vi "Gasteiler_Endpunkt.vi"   [LabVIEW 2020, in "Linearisierung v2.lvlib"]
uses:
  Linearisierung v2.lvlib
  Gasteiler/Aktionen FGV Gasteiler Daten.ctl
  Gasteiler/AK-Komm Gasteiler/Aktionen AK Komm.ctl
  Gasteiler/AK-Komm Gasteiler/Alter Gasteiler/Aktionen AK Komm_ALT.ctl
  Gasteiler/Horiba/Aktion Befehl.ctl
  Gasteiler/HovaCAL_Interface/Kommunikation/Aktion_FGV_HovaCAL_Interface_SetData.ctl
  Gasteiler/AK-Komm Gasteiler/AK Komm Gasteiler.lvlib
  Gasteiler/Horiba/Horiba GDC.lvlib
  Gasteiler/AK-Komm Gasteiler/Alter Gasteiler/Alter Gasteiler.lvlib
  Gasteiler/Gasteiler.lvlib
  Gasteiler/HovaCAL_Interface/Kommunikation/Kommunikation.lvlib
types:
  T1 = typedef "Linearisierung v2.lvlib/Gasteiler.lvlib/Aktionen FGV Gasteiler Daten.ctl" = enum16{"lesen", "Gasteiler Daten", "Seriellen Param.", "MB-Endwert", "laden", "speichern", "Anforderung", "TCP", "Aufzeichnung Start"}
  T2 = typedef "Linearisierung v2.lvlib/Gasteiler.lvlib/Gasteiler Daten.ctl" = cluster{"Gasteiler":T3, "Gasteiler Stufen":T4, "Gasteiler Type":T5, "Konfig Gasteiler":T6, "Gasteiler Span Eingänge":u16}
  T3 = typedef "String - Eingabefeld.ctl" = string
  T4 = typedef "Linearisierung v2.lvlib/Gasteiler.lvlib/Gasteiler Stufen.ctl" = u16
  T5 = typedef "Linearisierung v2.lvlib/GasteilerType.ctl" = u16
  T6 = typedef "System Einstellungen V2.lvlib/Gasteiler Auswahl.ctl" = u16
  T7 = typedef "Linearisierung v2.lvlib/Gasteiler.lvlib/AK Komm Gasteiler.lvlib/Aktionen AK Komm.ctl" = enum16{"lesen", "initialisieren", "beenden", "Status", "SMAN", "SREM", "STBY", "ASTF", "ASTZ", "SLST", "AGAT", "EGAK", "AGAK", "AKAK", "ADRU", "SKOP", "SVSA", "SVSZ", "SONO", "SAIR", "SNOX", "ANOX", "SSPL", "SRUC", "SLIN", "ALST", "ETYP", "SVIO", "LCYL", "CCYL", "DCYL", "SCYL", "GCYL", "DRGV", "DRDC"}
  T8 = typedef "Linearisierung v2.lvlib/Gasteiler.lvlib/AK Komm Gasteiler.lvlib/Alter Gasteiler.lvlib/Aktionen AK Komm_ALT.ctl" = enum16{"lesen", "initialisieren", "beenden", "SRES", "STBY", "SREM", "SMAN", "SLIN", "SLCH", "SLST", "SSPL", "AGAT", "ALST", "ASTZ", "ASTF", "AGAK", "EGAK"}
  T9 = typedef "Linearisierung v2.lvlib/Gasteiler.lvlib/Horiba GDC.lvlib/Aktion Befehl.ctl" = enum16{"lesen", "initialisieren", "Beenden", "Standby", "GD/CC", "Info", "Flow", "Alarm", "GD parameter", "GD point", "Durchfluss", "Spuelen1", "Spuelen1 On", "Spuelen1Off", "Spuelen2", "Ventil-Abfrage", "Reset"}
  T10 = typedef "Linearisierung v2.lvlib/Gasteiler.lvlib/HovaCAL_Interface.lvlib/Kommunikation.lvlib/Aktion_FGV_HovaCAL_Interface_SetData.ctl" = enum16{"lesen", "Konzentrationen", "Pumpen Parameter", "Pumpe Konzentration", "Pumpe run", "Temperaturen", "Fluss", "Limits", "init"}
  T11 = cluster{"input concentration setpoint":dbl, "output concentration setpoint":dbl}[]
  T12 = cluster{"input concentration setpoint":dbl, "output concentration setpoint":dbl}
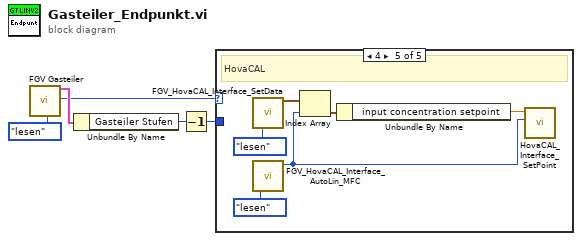
[diagram p0: block diagram]
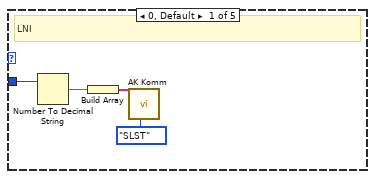
[diagram p2: hidden frame]
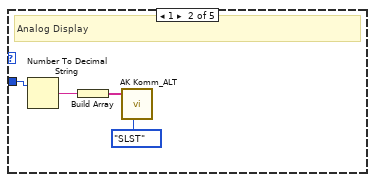
[diagram p3: hidden frame]
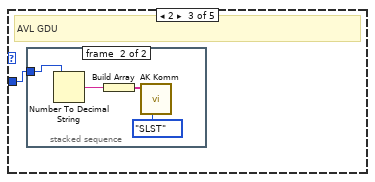
[diagram p4: hidden frame]
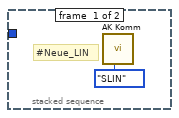
[diagram p5: hidden frame]
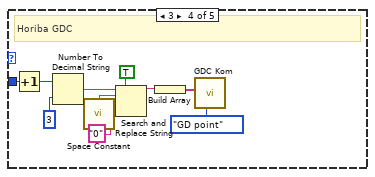
[diagram p6: hidden frame]
diagram:
  n1 = call "FGV Gasteiler.vi"("Aktionen"=Aktionen_FGV_Gasteiler_Daten."lesen") -> ("Gasteiler Daten"=w4:T2, "Gasteiler Type"=w2:T5)  [unwired: 11 in, 6 out]
  n2 = Unbundle By Name(w4) -> ("Gasteiler Stufen"=w1:T4)
  n3 = Decrement(x=w1) -> (x-1=w5:T4)
  n4 = case shown="4" w2 {
    tunnel: w5 -> [w6 w12 w14 w21 _]
    frame 0, Default {
      # "LNI"
      n5 = Number To Decimal String(number=w6) -> (decimal integer string=w9:string)  [unwired: 1 in]
      n6 = Build Array(w9) -> (w8:string[])
      n7 = call "AK Komm.vi"("Aktionen"=Aktionen_AK_Komm."SLST", "Daten"=w8) -> ()  [unwired: 3 in, 7 out]
    }
    frame 1 {
      # "Analog Display"
      n8 = Number To Decimal String(number=w12) -> (decimal integer string=w13:string)  [unwired: 1 in]
      n9 = Build Array(w13) -> (w11:string[])
      n10 = call "AK Komm_ALT.vi"("Aktionen_ALT"=Aktionen_AK_Komm_ALT."SLST", "Daten"=w11) -> ()  [unwired: 5 in, 5 out]
    }
    frame 2 {
      # "AVL GDU"
      n11 = stacked-sequence {
        tunnel: w14 -> [_ w18]
        frame #0 {
          # "#Neue_LIN"
          n12 = call "AK Komm.vi"("Aktionen"=Aktionen_AK_Komm."SLIN") -> ()  [unwired: 4 in, 7 out]
        }
        frame #1 {
          n13 = Number To Decimal String(number=w18) -> (decimal integer string=w19:string)  [unwired: 1 in]
          n14 = Build Array(w19) -> (w17:string[])
          n15 = call "AK Komm.vi"("Aktionen"=Aktionen_AK_Komm."SLST", "Daten"=w17) -> ()  [unwired: 3 in, 7 out]
        }
      }
    }
    frame 3 {
      # "Horiba GDC"
      n16 = Increment(x=w21) -> (x+1=w20:T4)
      n17 = Number To Decimal String(number=w20, width (-)=i16 3 ("Breite (-)")) -> (decimal integer string=w23:string)
      n18 = call <vilib>:"Space Constant.vi"() -> ("String"=w27:string)
      n19 = Search and Replace String(replace all?=TRUE ("Alle ersetzen? (F)"), input string=w23, search string=w27, replace string="0" ("Ersetzungs-String (\"\")")) -> (result string=w24:string)  [unwired: 4 in, 3 out]
      n20 = Build Array(w24) -> (w28:string[])
      n21 = call "GDC Kom.vi"("Befehl"=Aktion_Befehl."GD point", "Daten"=w28) -> ()  [unwired: 3 in, 7 out]
    }
    frame 4 {
      # "HovaCAL"
      n22 = call "FGV_HovaCAL_Interface_SetData.vi"("Aktion"=Aktion_FGV_HovaCAL_Interface_SetData."lesen") -> ("Set Values Cluster out"=w33:T11)  [unwired: 8 in, 6 out]
      n23 = call "FGV_HovaCAL_Interface_AutoLin_MFC.vi"("Aktion"=enum16{"lesen", "schreiben"}."lesen") -> ("AutoLin MFC out"=w32:u16)  [unwired: 7 in, 3 out]
      n24 = Index Array(array=w33, index=w32) -> (element=w31:T12)
      n25 = Unbundle By Name(w31) -> ("input concentration setpoint"=w30:dbl)
      n26 = call "HovaCAL_Interface_SetPoint.vi"("AutoLin MFC Index"=w32, "Konzentration"=w30) -> ()  [unwired: 9 in, 1 out]
    }
  }
